vi "Open Drive Motors.vi"(5 "Open Butterfly Drive?":bool, 6 "Idle Mode":T1, 7 "Set Master/Follower?":bool, 9 "CAN IDs":u8[](array[numeric]), 11 "Full Acceleration Time":sgl) -> ()   [LabVIEW 2018]
uses:
  <vilib>/Rock Robotics/WPI/ThirdParty/REV Robotics/SPARK MAX/Typedef/Spark MAX Idle Mode.ctl
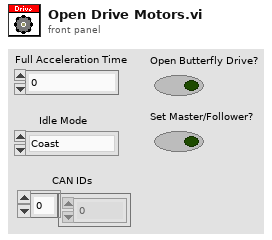
[diagram p1: front panel]
types:
  T1 = typedef "Spark MAX Idle Mode.ctl" = enum16{"Coast", "Brake"}
  T2 = typedef "WPI_MotorControlDeviceRef.ctl" = cluster{"DeviceStatus":errorcluster, "Type":T3, "PWM":cluster{"PWM Channel":T4, "DeadBand":T5}, "CAN":cluster{"Device Number":u8, "SetOutput VI Ref":variant, "GetOutput VI Ref":variant, "Enable VI Ref":variant, "Disable VI Ref":variant, "Data":variant}, "Invert":bool, "DIO PWM":cluster{"PWM \"Enable\" Channel":T4, "DIOChannel":T6, "PWM Rate":dbl}}
  T3 = typedef "WPI_MotorControlType.ctl" = enum16{"PWM", "CAN", "DIO PWM"}
  T4 = typedef "FPGA_DIOPWMChannel.ctl" = enum8{"PWM 0", "PWM 1", "PWM 2", "PWM 3", "PWM 4", "PWM 5", "PWM 6", "PWM 7", "PWM 8", "PWM 9", "PWM MXP 0", "PWM MXP 1", "PWM MXP 2", "PWM MXP 3", "PWM MXP 4", "PWM MXP 5", "PWM MXP 6", "PWM MXP 7", "PWM MXP 8", "PWM MXP 9", "Invalid"}
  T5 = typedef "WPI_PWMDeadband.ctl" = cluster{"Name":string, "maxPositivePwm":i32, "minPositivePwm":i32, "centerPwm":i32, "maxNegativePwm":i32, "minNegativePwm":i32, "angularRange":u16}
  T6 = typedef "FPGA_DIOChannel.ctl" = enum8{"DIO 0", "DIO 1", "DIO 2", "DIO 3", "DIO 4", "DIO 5", "DIO 6", "DIO 7", "DIO 8", "DIO 9", "DIO MXP 0", "DIO MXP 1", "DIO MXP 2", "DIO MXP 3", "DIO MXP 4", "DIO MXP 5", "DIO MXP 6", "DIO MXP 7", "DIO MXP 8", "DIO MXP 9", "DIO MXP 10", "DIO MXP 11", "DIO MXP 12", "DIO MXP 13", "DIO MXP 14", "DIO MXP 15", "SPI Port CS1", "SPI Port CS2", "SPI Port CS3", "SPI Port MISO", "SPI Port MOSI", "Invalid"}
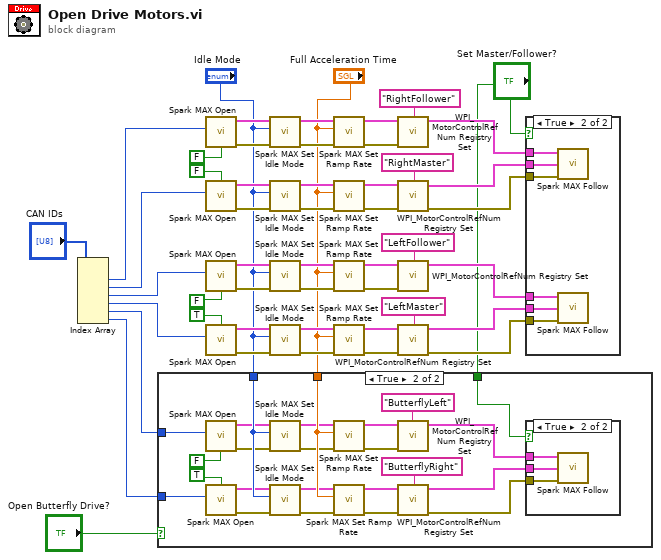
[diagram p0: block diagram]
diagram:
  n1 = Index Array(array="CAN IDs") -> (element #1=w11:u8, element #2=w10:u8, element #3=w9:u8, element #4=w8:u8, element #5=w7:u8, element #6=w6:u8)  [unwired: 6 in]
  n2 = case shown="True" "Open Butterfly Drive?" {
    tunnel: w7 -> [_ w73]
    tunnel: w6 -> [_ w72]
    tunnel: "Full Acceleration Time" -> [_ w71]
    tunnel: "Idle Mode" -> [_ w70]
    tunnel: "Set Master/Follower?" -> [_ w50]
    frame False {
    }
    frame True {
      n3 = call <vilib>:"Spark MAX Open.vi"("Invert"=FALSE, "Device Number"=w73) -> ("error out"=w54:errorcluster, "MotorControlDeviceRef"=w56:T2)  [unwired: 8 in]
      n4 = call <vilib>:"Spark MAX Open.vi"("Invert"=TRUE, "Device Number"=w72) -> ("error out"=w53:errorcluster, "MotorControlDeviceRef"=w55:T2)  [unwired: 8 in]
      n5 = call <vilib>:"Spark MAX Set Idle Mode.vi"("error in (no error)"=w54, "Idle Mode"=w70, "MotorControlDeviceRef in"=w56) -> ("error out"=w62:errorcluster, "MotorControlDeviceRef out"=w63:T2)  [unwired: 7 in]
      n6 = call <vilib>:"Spark MAX Set Idle Mode.vi"("error in (no error)"=w53, "Idle Mode"=w70, "MotorControlDeviceRef in"=w55) -> ("error out"=w60:errorcluster, "MotorControlDeviceRef out"=w64:T2)  [unwired: 7 in]
      n7 = call <vilib>:"Spark MAX Set Ramp Rate.vi"("error in (no error)"=w62, "Seconds from neutral to full (0)"=w71, "MotorControlDeviceRef in"=w63) -> ("error out"=w61:errorcluster, "MotorControlDeviceRef"=w65:T2)  [unwired: 7 in]
      n8 = call <vilib>:"Spark MAX Set Ramp Rate.vi"("error in (no error)"=w60, "Seconds from neutral to full (0)"=w71, "MotorControlDeviceRef in"=w64) -> ("error out"=w59:errorcluster, "MotorControlDeviceRef"=w66:T2)  [unwired: 7 in]
      n9 = call <vilib>:"WPI_MotorControlRefNum Registry Set.vi"("error in (no error)"=w61, "refnum name"="ButterflyLeft", "MotorControlDevRef"=w65) -> ("MotorControlDevRef"=w69:T2)  [unwired: 7 in, 1 out]
      n10 = call <vilib>:"WPI_MotorControlRefNum Registry Set.vi"("error in (no error)"=w59, "refnum name"="ButterflyRight", "MotorControlDevRef"=w66) -> ("error out"=w67:errorcluster, "MotorControlDevRef"=w68:T2)  [unwired: 7 in]
      n11 = case shown="True" w50 {
        tunnel: w69 -> [_ w76]
        tunnel: w68 -> [_ w75]
        tunnel: w67 -> [_ w74]
        frame False {
        }
        frame True {
          n12 = call <vilib>:"Spark MAX Follow.vi"("error in (no error)"=w74, "Master Controller"=w75, "MotorControlDeviceRef"=w76) -> ()  [unwired: 7 in, 2 out]
        }
      }
    }
  }
  n13 = call <vilib>:"Spark MAX Open.vi"("Invert"=FALSE, "Device Number"=w11) -> ("error out"=w36:errorcluster, "MotorControlDeviceRef"=w41:T2)  [unwired: 8 in]
  n14 = call <vilib>:"Spark MAX Open.vi"("Invert"=FALSE, "Device Number"=w10) -> ("error out"=w34:errorcluster, "MotorControlDeviceRef"=w40:T2)  [unwired: 8 in]
  n15 = call <vilib>:"Spark MAX Open.vi"("Invert"=FALSE, "Device Number"=w9) -> ("error out"=w32:errorcluster, "MotorControlDeviceRef"=w42:T2)  [unwired: 8 in]
  n16 = call <vilib>:"Spark MAX Open.vi"("Invert"=TRUE, "Device Number"=w8) -> ("error out"=w30:errorcluster, "MotorControlDeviceRef"=w43:T2)  [unwired: 8 in]
  n17 = call <vilib>:"Spark MAX Set Idle Mode.vi"("error in (no error)"=w36, "Idle Mode"="Idle Mode", "MotorControlDeviceRef in"=w41) -> ("error out"=w35:errorcluster, "MotorControlDeviceRef out"=w38:T2)  [unwired: 7 in]
  n18 = call <vilib>:"Spark MAX Set Idle Mode.vi"("error in (no error)"=w34, "Idle Mode"="Idle Mode", "MotorControlDeviceRef in"=w40) -> ("error out"=w33:errorcluster, "MotorControlDeviceRef out"=w39:T2)  [unwired: 7 in]
  n19 = call <vilib>:"Spark MAX Set Idle Mode.vi"("error in (no error)"=w32, "Idle Mode"="Idle Mode", "MotorControlDeviceRef in"=w42) -> ("error out"=w27:errorcluster, "MotorControlDeviceRef out"=w45:T2)  [unwired: 7 in]
  n20 = call <vilib>:"Spark MAX Set Idle Mode.vi"("error in (no error)"=w30, "Idle Mode"="Idle Mode", "MotorControlDeviceRef in"=w43) -> ("error out"=w29:errorcluster, "MotorControlDeviceRef out"=w44:T2)  [unwired: 7 in]
  n21 = call <vilib>:"Spark MAX Set Ramp Rate.vi"("error in (no error)"=w35, "Seconds from neutral to full (0)"="Full Acceleration Time", "MotorControlDeviceRef in"=w38) -> ("error out"=w25:errorcluster, "MotorControlDeviceRef"=w47:T2)  [unwired: 7 in]
  n22 = call <vilib>:"Spark MAX Set Ramp Rate.vi"("error in (no error)"=w33, "Seconds from neutral to full (0)"="Full Acceleration Time", "MotorControlDeviceRef in"=w39) -> ("error out"=w26:errorcluster, "MotorControlDeviceRef"=w46:T2)  [unwired: 7 in]
  n23 = call <vilib>:"Spark MAX Set Ramp Rate.vi"("error in (no error)"=w27, "Seconds from neutral to full (0)"="Full Acceleration Time", "MotorControlDeviceRef in"=w45) -> ("error out"=w31:errorcluster, "MotorControlDeviceRef"=w48:T2)  [unwired: 7 in]
  n24 = call <vilib>:"Spark MAX Set Ramp Rate.vi"("error in (no error)"=w29, "Seconds from neutral to full (0)"="Full Acceleration Time", "MotorControlDeviceRef in"=w44) -> ("error out"=w28:errorcluster, "MotorControlDeviceRef"=w49:T2)  [unwired: 7 in]
  n25 = call <vilib>:"WPI_MotorControlRefNum Registry Set.vi"("error in (no error)"=w25, "refnum name"="RightFollower" ("string"), "MotorControlDevRef"=w47) -> ("MotorControlDevRef"=w19:T2)  [unwired: 7 in, 1 out]
  n26 = call <vilib>:"WPI_MotorControlRefNum Registry Set.vi"("error in (no error)"=w26, "refnum name"="RightMaster", "MotorControlDevRef"=w46) -> ("error out"=w3:errorcluster, "MotorControlDevRef"=w18:T2)  [unwired: 7 in]
  n27 = call <vilib>:"WPI_MotorControlRefNum Registry Set.vi"("error in (no error)"=w31, "refnum name"="LeftFollower", "MotorControlDevRef"=w48) -> ("MotorControlDevRef"=w15:T2)  [unwired: 7 in, 1 out]
  n28 = call <vilib>:"WPI_MotorControlRefNum Registry Set.vi"("error in (no error)"=w28, "refnum name"="LeftMaster", "MotorControlDevRef"=w49) -> ("error out"=w21:errorcluster, "MotorControlDevRef"=w17:T2)  [unwired: 7 in]
  n29 = case shown="True" "Set Master/Follower?" {
    tunnel: w21 -> [_ w82]
    tunnel: w19 -> [_ w81]
    tunnel: w18 -> [_ w80]
    tunnel: w17 -> [_ w79]
    tunnel: w15 -> [_ w78]
    tunnel: w3 -> [_ w77]
    frame False {
    }
    frame True {
      n30 = call <vilib>:"Spark MAX Follow.vi"("error in (no error)"=w77, "Master Controller"=w80, "MotorControlDeviceRef"=w81) -> ()  [unwired: 7 in, 2 out]
      n31 = call <vilib>:"Spark MAX Follow.vi"("error in (no error)"=w82, "Master Controller"=w79, "MotorControlDeviceRef"=w78) -> ()  [unwired: 7 in, 2 out]
    }
  }
